vi "updateInicatorsMainVi.vi"(6 "Data String out":string, 7 "Boolean":bool, 9 "Array":refnum<vi>[](array[refnum]), 10 "Channel Selector":string, 11 "error in":errorcluster) -> (0 "Data String out 2":string, 2 "name/data":string[][](array[string]), 3 "error out":errorcluster)   [LabVIEW 2020]
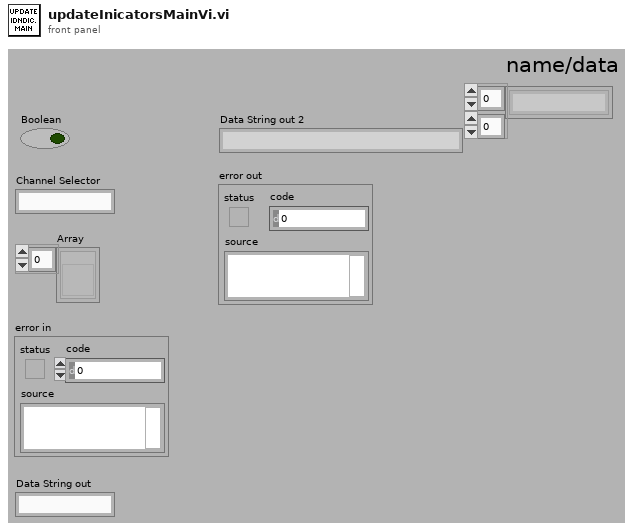
[diagram p1: front panel]
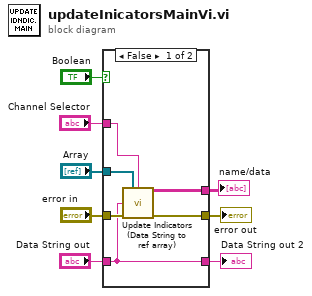
[diagram p0: block diagram]
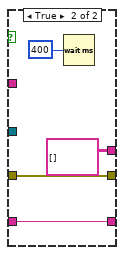
[diagram p2: hidden frame]
diagram:
  n1 = case shown="False" "Boolean" {
    tunnel: "Array" -> [w13 _]
    tunnel: "error in" -> [w12 w18]
    tunnel: [w14 w18] -> w3
    tunnel: "Channel Selector" -> [w10 _]
    tunnel: [w11 w16] -> w6
    tunnel: "Data String out" -> [w11 w16]
    tunnel: [w9 string[][] [] ("name/data")] -> w1
    frame False {
      n2 = call "Update Indicators (Data String to ref array).vi"("Array"=w13, "Active Channel"=w10, "Data String"=w11, "error in (no error)"=w12) -> ("name/data"=w9:string[][], "error out"=w14:errorcluster)  [unwired: 10 in]
    }
    frame True {
      n3 = Wait (ms)(milliseconds to wait=u32 400) -> ()  [unwired: 1 out]
    }
  }
  "Data String out 2" <- w6
  "error out" <- w3
  "name/data" <- w1
